vi "ConnectionDied.vi"(8 "error in (no error)":errorcluster, 10 "Connection":refnum<class "Connection.lvclass">, 11 "Tcp in":refnum<class "Tcp.lvclass">) -> (0 "error out":errorcluster, 3 "Tcp out":refnum<class "Tcp.lvclass">)   [LabVIEW 2022 SP3, in "Tcp.lvlib" / "Tcp.lvclass"]
uses:
  Tcp.lvclass
  TcpSocket/Source/TcpSocket/Connection/Connection.lvclass
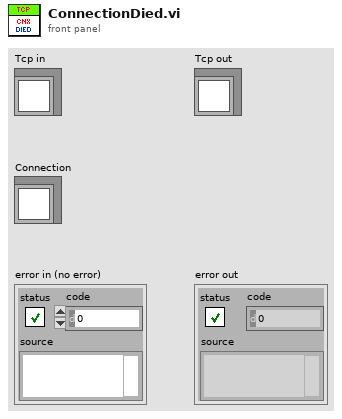
[diagram p1: front panel]
types:
  T1 = map{u64, refnum<class "Message Enqueuer.lvclass">}
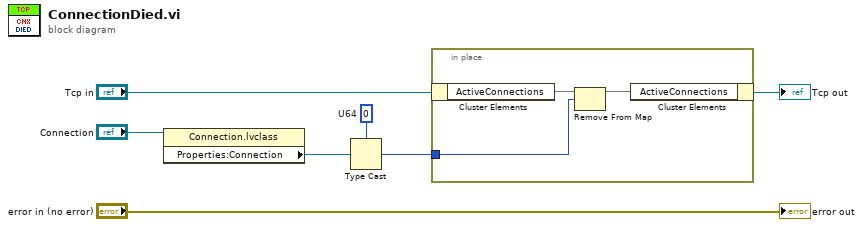
[diagram p0: block diagram]
diagram:
  w1 = u64 0  # U64
  n1 = property class="Connection.lvclass"(reference="Connection") -> ("Properties:Connection"=w4:refnum<k5>)  [unwired: 1 in, 2 out]
  n2 = Type Cast(type=w1, x=w4) -> (*(type *) &x=w2:u64)
  n3 = in-place {
    in-place-border: w2 -> [w8]
    n4 = in-place-cluster #1("Tcp in") -> ("ActiveConnections"=w10:T1)
    n5 = Remove From Map(10:w8, 11:w10) -> (3:w9:T1)  [unwired: 2 out]
    n6 = in-place-cluster #1("ActiveConnections"=w9) -> (→"Tcp out":refnum<class "Tcp.lvclass">)
  }
  "error out" <- "error in (no error)"
